vi "Process.vi"(8 "error in":errorcluster, 11 "Example Instrument UI":refnum<class "SR7220 UI.lvclass">) -> (0 "error out":errorcluster, 3 "Example Instrument UI out":refnum<class "SR7220 UI.lvclass">)   [LabVIEW 2016, in "SR7220 UI.lvclass"]
doc: "---------------------------------------------------------------\nJKI State Machine Objects™\nhttp://jki.net/state-machine-objects/\nCopyright (C) 2005-2015, JKI <info@jki.net>\nALL RIGHTS RESERVEDJKI State Machine Objects (SMO) 1.0.0.5\nJKI - JKI\nCopyright (c) 2016, JKI"
uses:
  SR7220 UI.lvclass
  C:/Program Files (x86)/National Instruments/LabVIEW 2016/vi.lib/JKI/JKI SMO/SMO/SMO.lvclass
  C:/Program Files (x86)/National Instruments/LabVIEW 2016/vi.lib/JKI/JKI SMO/SMO.UI/SMO.UI.lvclass
  Instrument.SR7270/Typedefs/SignalChannelConfig--Cluster.ctl
  Instrument.SR7270/Driver/Typedefs/VMODE--enum.ctl
  Instrument.SR7270/Driver/Typedefs/FLOAT--enum.ctl
  Instrument.SR7270/Driver/Typedefs/FET--enum.ctl
  Instrument.SR7270/Driver/Typedefs/LF--enum.ctl
  Instrument.SR7270/Driver/Typedefs/SEN-IMODE0--enum.ctl
  <vilib>/JKI/JKI SMO/SMO/Typedefs/Parent Call--Enum.ctl
  SR7220 UI.lvclass/SR7220 UI.ctl
  levylab_inst/lvsrc/SMOs/Instrument/Typedefs/PrivateEvents--Instrument.SendMessage.ctl
  <vilib>/JKI/JKI SMO/SMO.UI/SMO.UI.lvclass
  <vilib>/JKI/JKI SMO/SMO/SMO.lvclass
  levylab_inst/lvsrc/SMOs/Instrument/Instrument.lvclass
  Instrument.SR7270/Instrument.SR7270.lvclass
  Instrument.SR7270/Driver/SR7270 Drivers.lvclass
panel:
  out "Slide 4":dbl(slide) scale=0.0..10.0 scale format="%#_6p"
  out "Slide 3":dbl(slide) scale=0.0..10.0 scale format="%#_6p"
  out "Slide 2":dbl(slide) scale=0.0..10.0 scale format="%#_6p"
  out "Slide":dbl(slide) scale=0.0..10.0 scale format="%#_6p"
  in  "update time (ms)":u32=100
  out "Numeric 4":dbl
  out "Numeric 3":dbl
  out "Numeric 2":dbl
  out "Numeric":dbl
  in  "Display Type":enum16{"X", "Y", "MAG", "PHASE"}(ring)=enum."PHASE"
  in  "Display Type":enum16{"X", "Y", "MAG", "PHASE"}(ring)=enum."PHASE"
  in  "Display Type":enum16{"X", "Y", "MAG", "PHASE"}(ring)=enum."PHASE"
  in  "Display Type":enum16{"X", "Y", "MAG", "PHASE"}(ring)=enum."PHASE"
  in  "down":bool
  in  "up":bool
  in  "Sensitivity IMODE0":T1=enum."5 nV"
  in  "Signal Channel Config":T2={"Input Mode"=enum."Both Grounded", "Input Connector Shell"=enum."Float", "Input Device"=enum."FET", "Line Rejection Filter"=enum."Off"}
  in  "STOP":bool
  # "SMO UI Template"
  # "For instructions on how to use the JKI State Machine Objects, examples and video tutorials, visit:\nhttp://jki.net/state-machine-objects/\n\nJKI State Machine Objects™\nhttp://jki.net/state-machine-objects/\nCopyright (C) 2005-2015, JKI <info@jki.net>\nALL RIGHTS RESERVED"
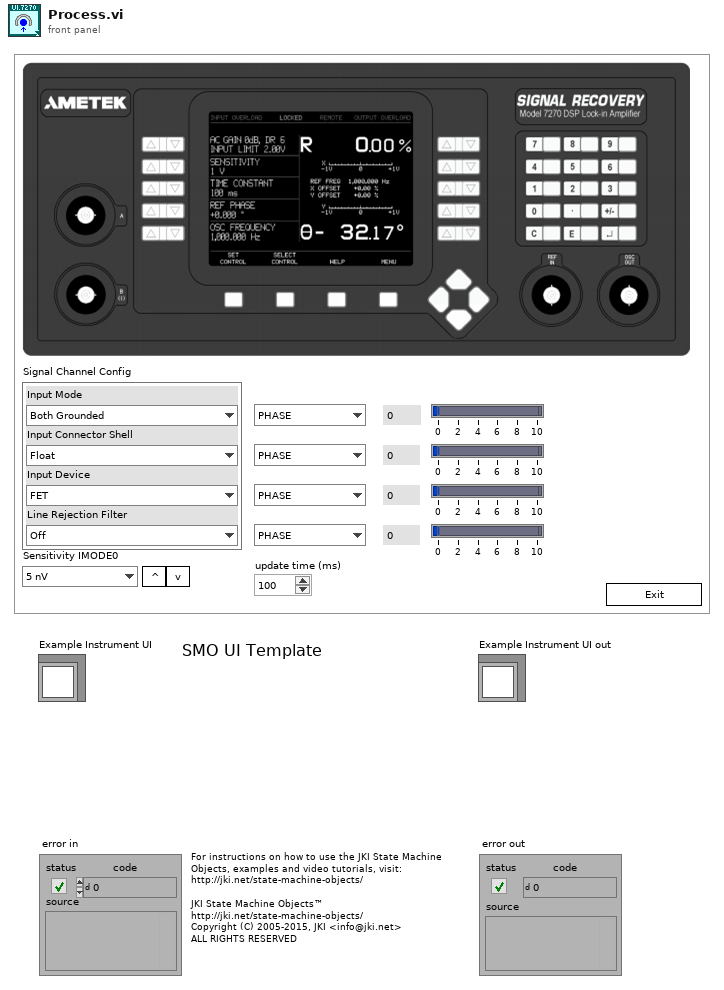
[diagram p1: front panel]
types:
  T1 = typedef "SR7270 Drivers.lvclass/SEN-IMODE0--enum.ctl" = enum16{"2 nV", "5 nV", "10 nV", "20 nV", "50 nV", "100 nV", "200 nV", "500 nV", "1 µV", "2 µV", "5 µV", "10 µV", "20 µV", "50 µV", "100 µV", "200 µV", "500 µV", "1 mV", "2 mV", "5 mV", "10 mV", "20 mV", "50 mV", "100 mV", "200 mV", "500 mV", "1 V"}
  T2 = typedef "Instrument.SR7270.lvclass/SignalChannelConfig--Cluster.ctl" = cluster{"Input Mode":T3, "Input Connector Shell":T4, "Input Device":T5, "Line Rejection Filter":T6}
  T3 = typedef "SR7270 Drivers.lvclass/VMODE--enum.ctl" = enum16{"Both Grounded", "A input only", "-B input only", "A-B differential"}
  T4 = typedef "SR7270 Drivers.lvclass/FLOAT--enum.ctl" = enum16{"Ground", "Float"}
  T5 = typedef "SR7270 Drivers.lvclass/FET--enum.ctl" = enum16{"Bipolar", "FET"}
  T6 = typedef "SR7270 Drivers.lvclass/LF--enum.ctl" = enum16{"Off", "60 Hz", "120 Hz", "60 & 120 Hz"}
  T7 = typedef "SMO.lvclass/Parent Call--Enum.ctl" = enum16{"Allows parent to run", "Does not request parent to run"}
  T8 = enum32{"invalid app kind", "Development System", "Run Time System", "Student Edition", "Embedded LabVIEW", "Evaluation", "Custom"}
  T9 = enum32{"Invalid", "Standard", "Closed", "Hidden", "Minimized", "Maximized"}
  T10 = typedef "Instrument.lvclass/PrivateEvents--Instrument.SendMessage.ctl" = cluster{"Message":cluster{"Command":string, "Data":variant}, "Message ID":u32}
  T11 = typedef "Instrument.lvclass/PublicEvents--Instrument.get all.ctl" = variant
  T12 = cluster{"Core":cluster{"Current VI Reference":refnum<vi>, "Close Panel on Exit?":bool, "error":errorcluster}, "Self Reference":refnum<class "SR7220 UI.lvclass">, "Instrument":refnum<class "Instrument.lvclass">, "getAll":variant, "Data":variant}
  T13 = cluster{"Current VI Reference":refnum<vi>, "Close Panel on Exit?":bool, "error":errorcluster}
  T14 = typedef "SMO.lvclass/Protected Events.ctl" = cluster{"StopProcesses":refnum<user-event>, "AbortProcesses":refnum<user-event>, "Config Changed":refnum<user-event>, "Dependency":refnum<user-event>}
  T15 = typedef "Instrument.lvclass/PublicEvents--Cluster.ctl" = cluster{"get all":refnum<user-event>}
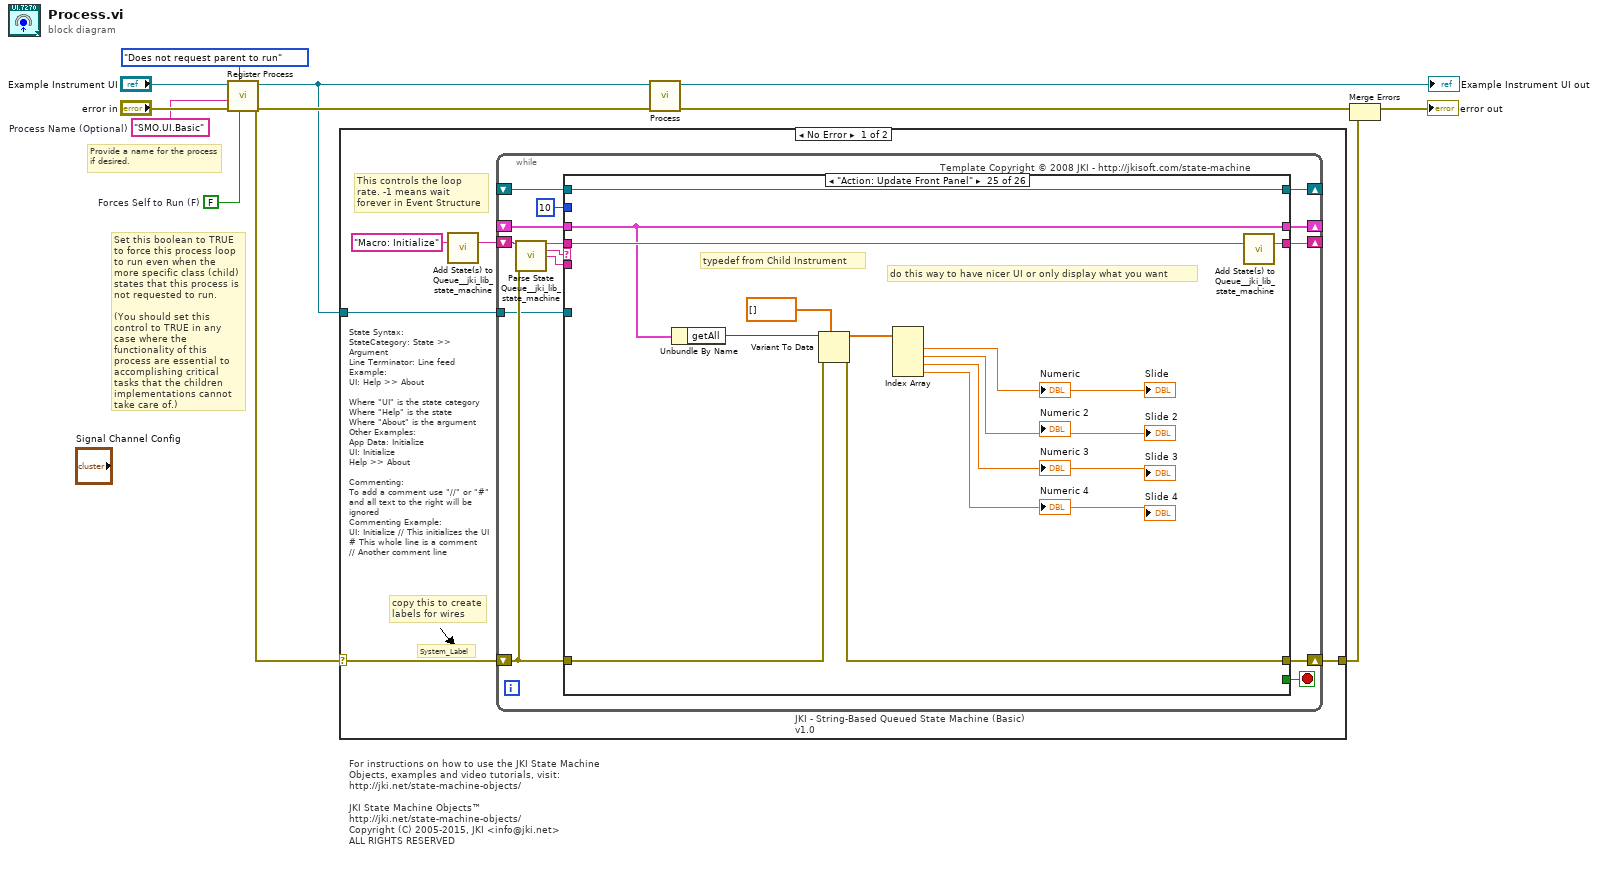
[diagram p0: block diagram]
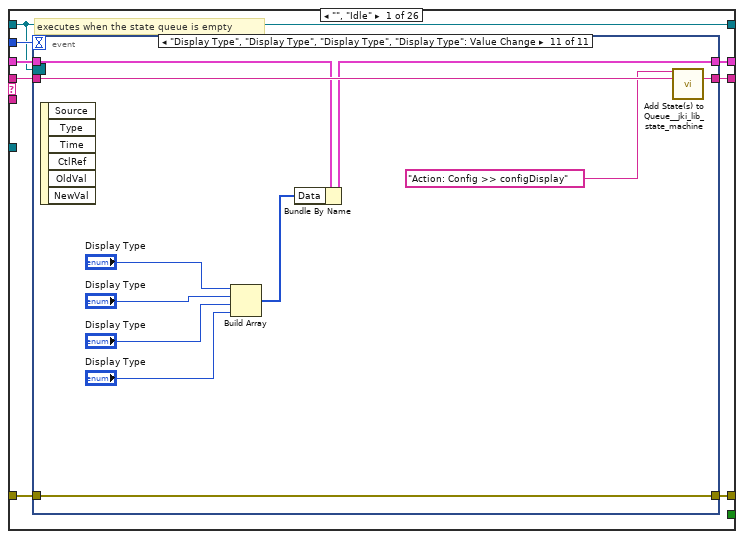
[diagram p2: hidden frame]
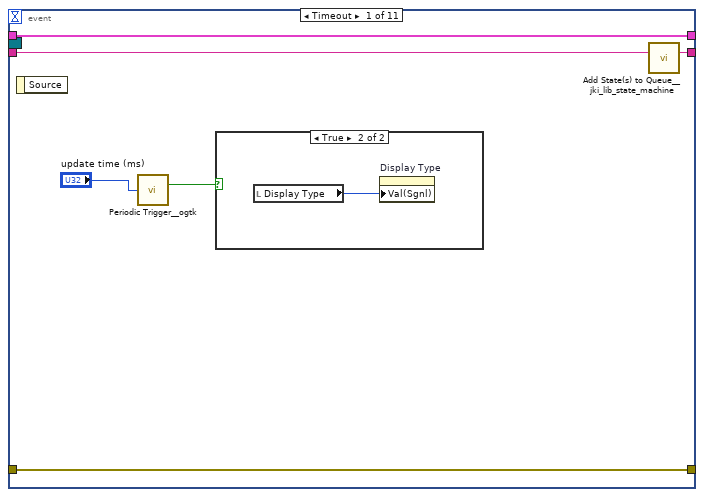
[diagram p3: hidden frame]
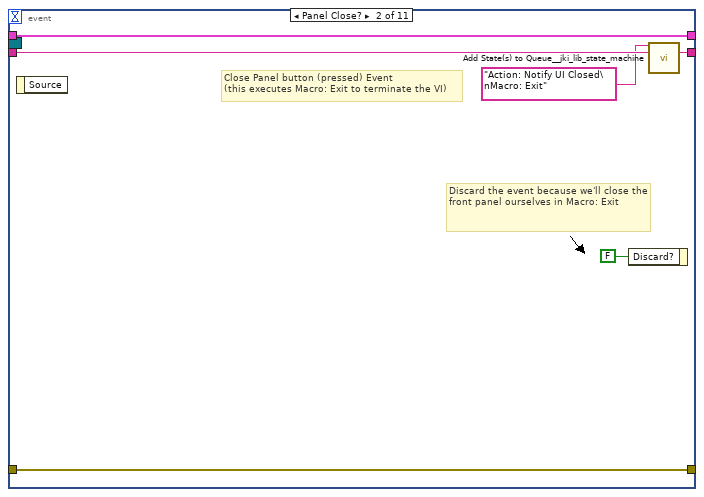
[diagram p5: hidden frame]
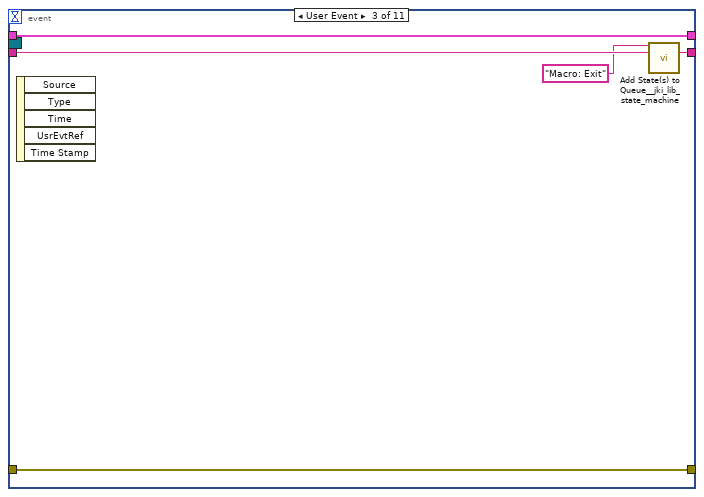
[diagram p6: hidden frame]
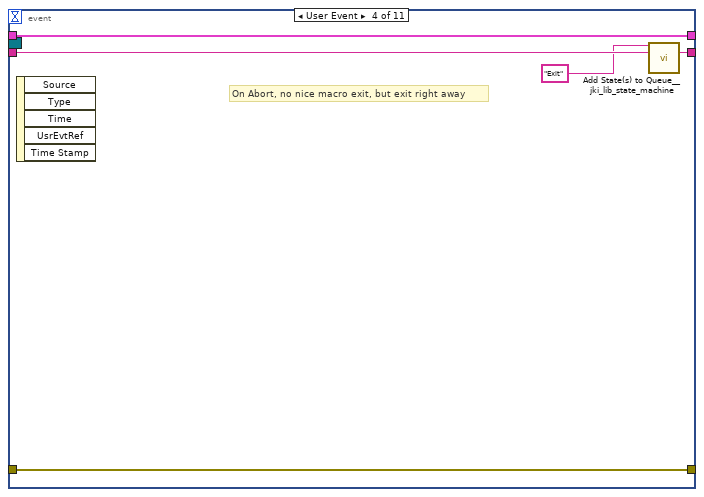
[diagram p7: hidden frame]
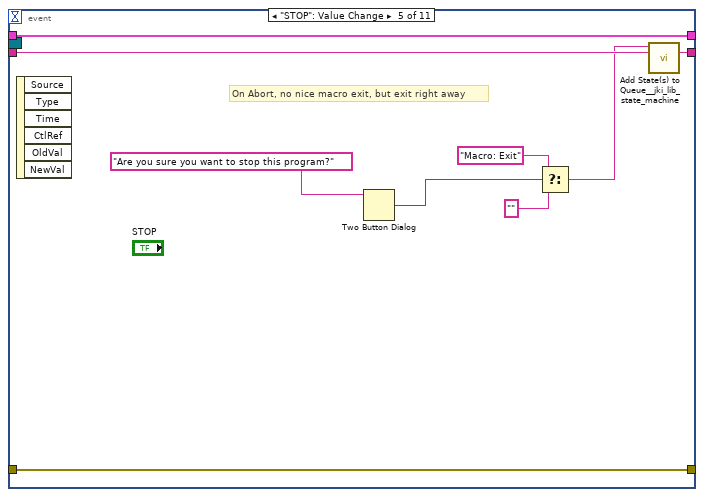
[diagram p8: hidden frame]
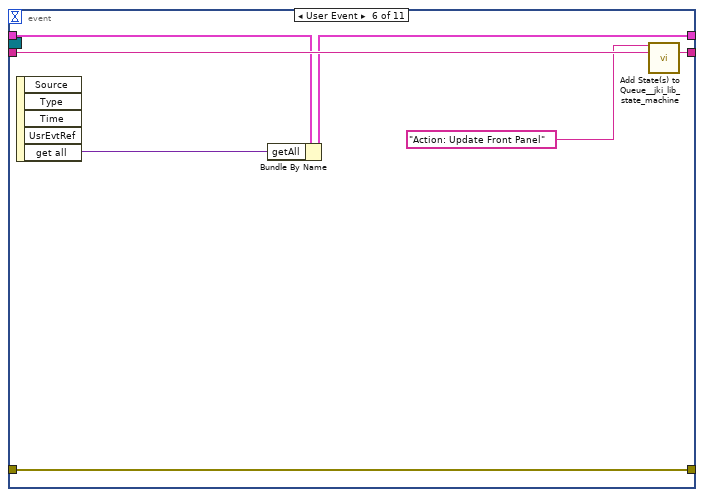
[diagram p9: hidden frame]
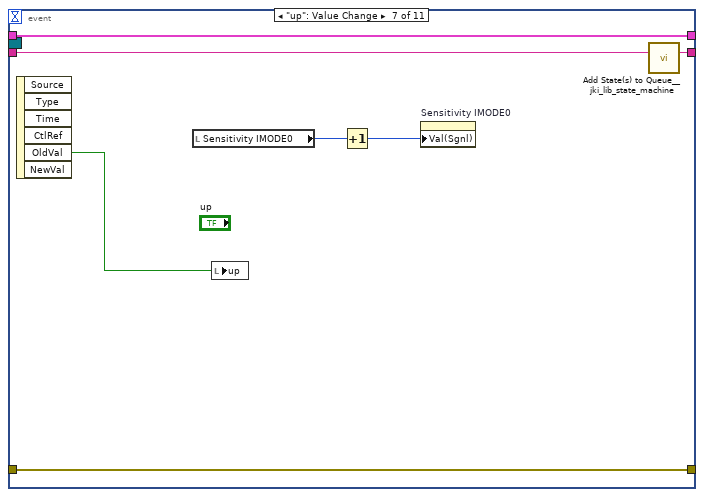
[diagram p10: hidden frame]
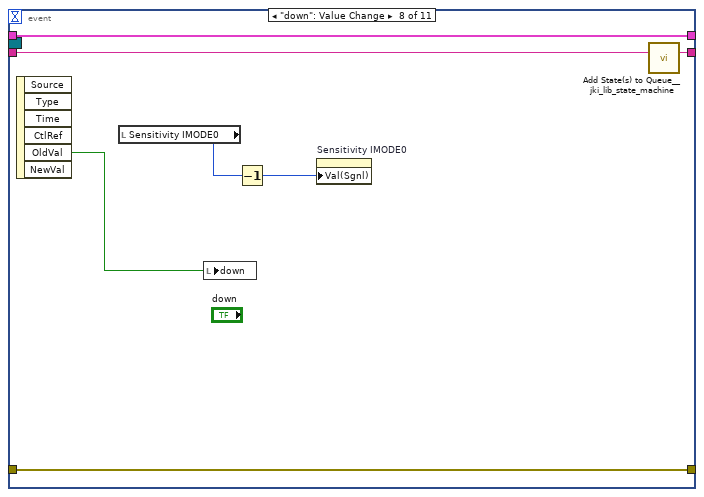
[diagram p11: hidden frame]
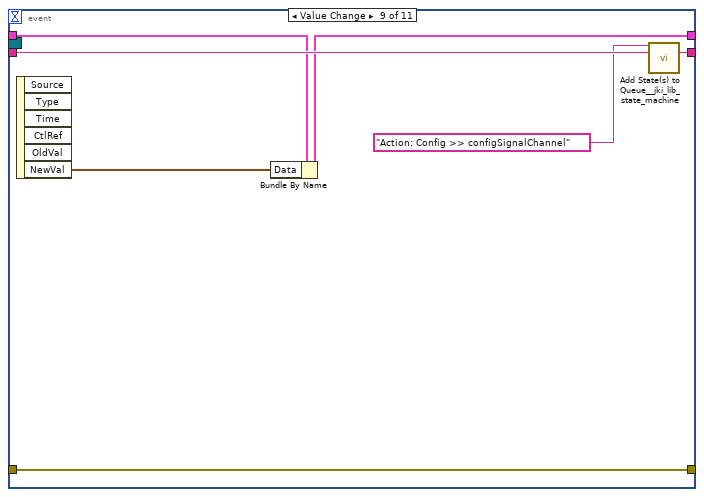
[diagram p12: hidden frame]
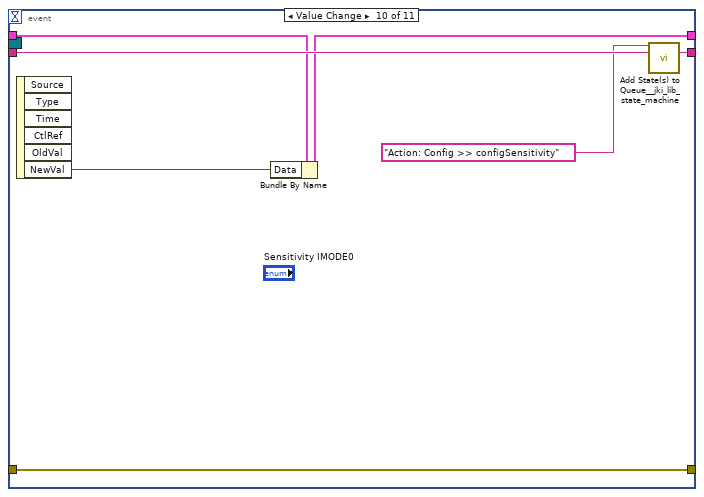
[diagram p13: hidden frame]
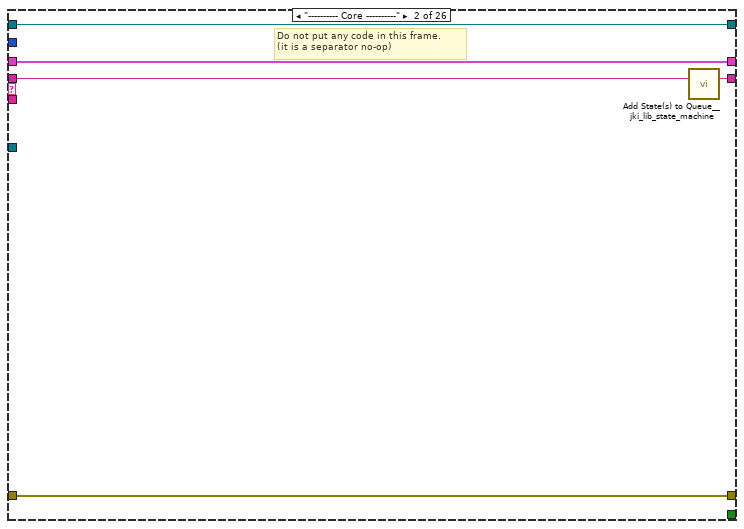
[diagram p14: hidden frame]
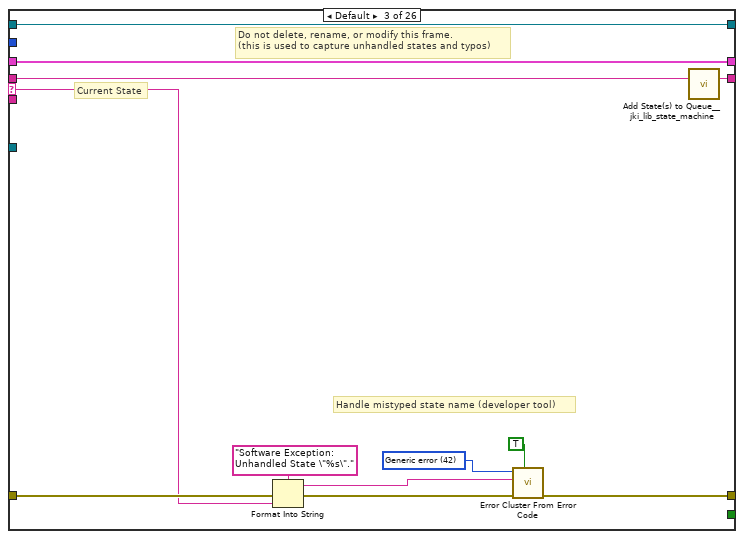
[diagram p15: hidden frame]
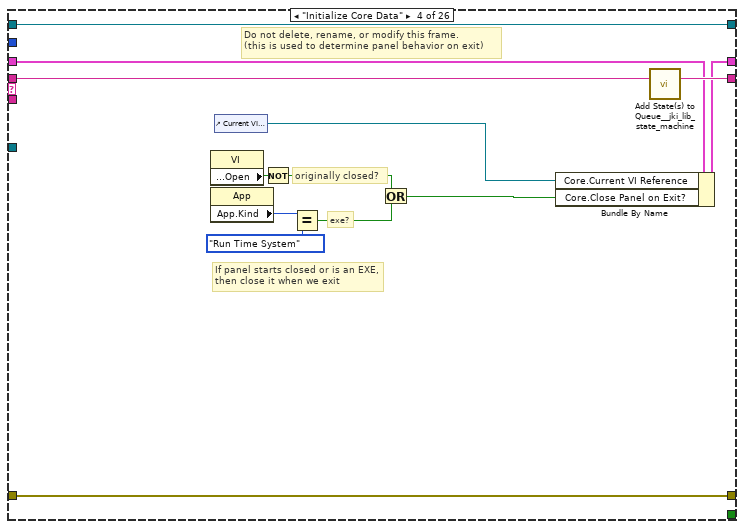
[diagram p16: hidden frame]
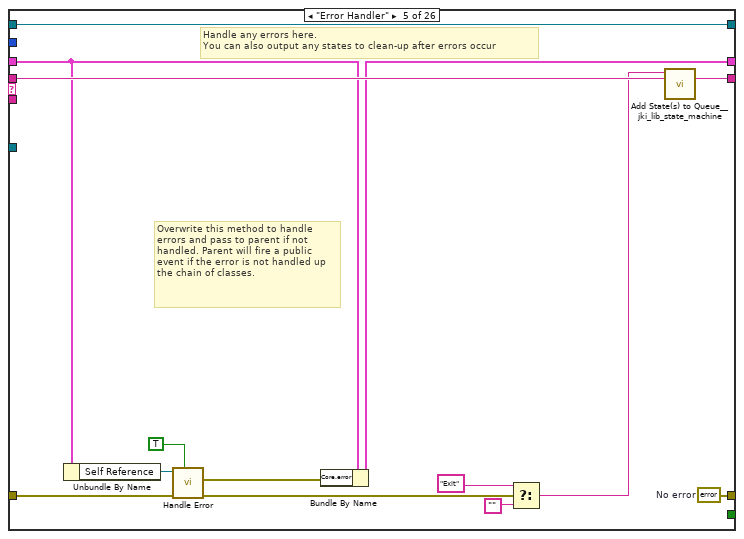
[diagram p17: hidden frame]
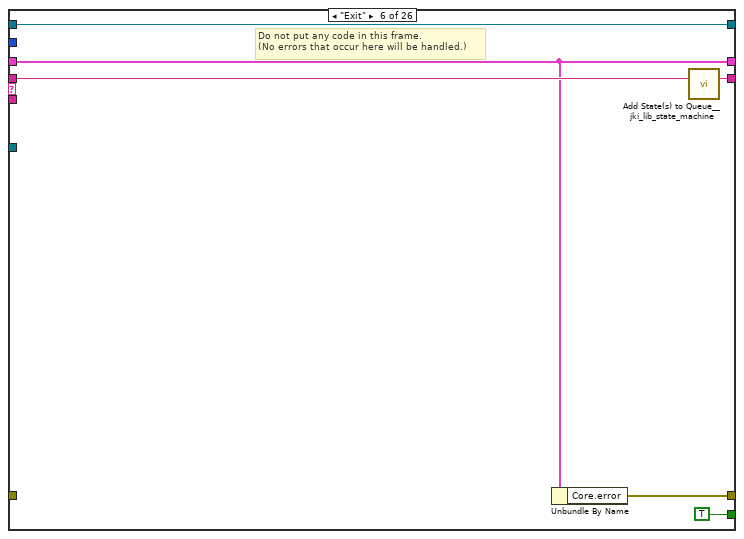
[diagram p18: hidden frame]
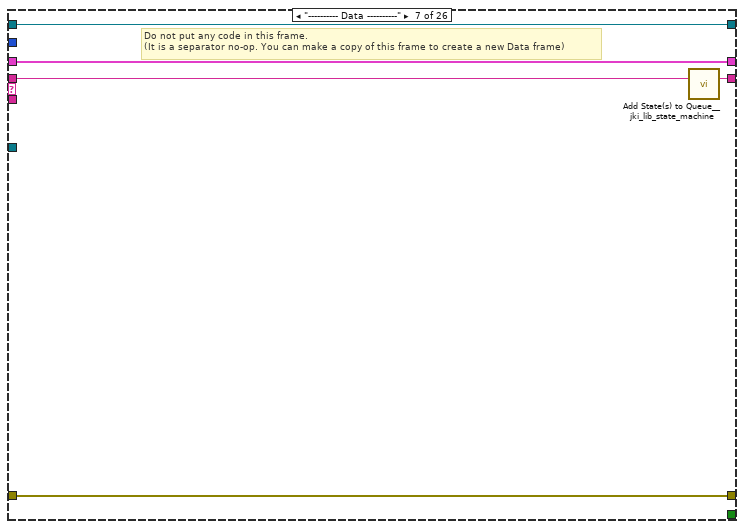
[diagram p19: hidden frame]
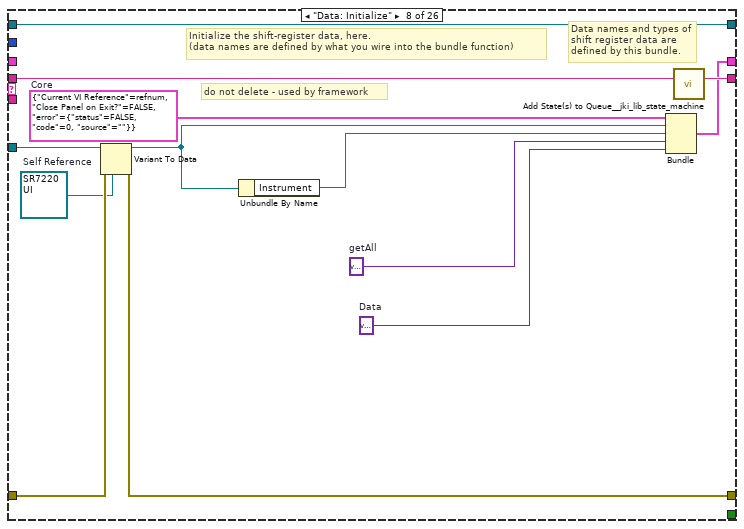
[diagram p20: hidden frame]
diagram:
  w2 = FALSE  # Forces Self to Run (F)
  w1 = "SMO.UI.Basic"  # Process Name (Optional)
  # "Provide a name for the process\nif desired."
  # "Set this boolean to TRUE to force this process loop to run even when the more specific class (child) states that this process is not requested to run.\n\n(You should set this control to TRUE in any case where the functionality of this process are essential to accomplishing critical tasks that the children implementations cannot take care of.)"
  # "For instructions on how to use the JKI State Machine Objects, examples and video tutorials, visit:\nhttp://jki.net/state-machine-objects/\n\nJKI State Machine Objects™\nhttp://jki.net/state-machine-objects/\nCopyright (C) 2005-2015, JKI <info@jki.net>\nALL RIGHTS RESERVED"
  n1 = call <vilib>:"Register Process.vi"("Forces Self to Run (F)"=w2, "Parent Call"=Parent_Call--Enum."Does not request parent to run", "error in (no error)"="error in", "Process Name (optional)"=w1, "SMO"="Example Instrument UI") -> ("error out"=w8:errorcluster, "SMO out"=w7:refnum<class "SR7220 UI.lvclass">)  [unwired: 5 in]
  n2 = case shown="No Error" w8 {
    selector: w8 -> [w13 w367]
    tunnel: w7 -> [w14 _]
    tunnel: [w12 w367] -> w4
    frame No Error {
      # "State Syntax:\nStateCategory: State >> Argument\nLine Terminator: Line feed\nExample:\nUI: Help >> About\n\nWhere \"UI\" is the state category\nWhere \"Help\" is the state\nWhere \"About\" is the argument\nOther Examples:\nApp Data: Initialize\nUI: Initialize\nHelp >> About\n\nCommenting:\nTo add a comment use \"//\" or \"#\" and all text to the right will be ignored\nCommenting Example:\nUI: Initialize // This initializes the UI\n# This whole line is a comment\n// Another comment line"
      # "copy this to create labels for wires"
      # "This controls the loop rate. -1 means wait forever in Event Structure"
      # "System_Label"
      n3 = call <vilib>:"Add State(s) to Queue__jki_lib_state_machine.vi"("State(s) in (\"\")"="Macro: Initialize") -> ("States Out"=w16:string)  [unwired: 14 in]
      n4 = while "JKI - String-Based Queued State Machine (Basic) v1.0" {
        shift-right: [w23] -> _
        shift-left: _ -> [w22]
        shift-right: [w26] -> w12
        shift-left: w13 -> [w20]
        shift-right: [w25] -> _
        shift-left: w16 -> [w27]
        tunnel: w14 -> [w19]
        shift-right: [w18] -> _
        shift-left: _ -> [w17]
        stop <- w24 stop-if-true
        # "Template Copyright © 2008 JKI - http://jkisoft.com/state-machine"
        n5 = call <vilib>:"Parse State Queue__jki_lib_state_machine.vi"("State Queue"=w27, "Error In (no error)"=w20) -> ("Remaining States"=w29:string, "Current State"=w30:string, "Arguments"=w28:string)  [unwired: 11 in]
        n6 = case shown="\"Action: Update Front Panel\"" w30 {
          selector: w30 -> [_ _ w123 _ _ _ _ _ _ _ _ _ _ _ _ _ _ _ _ _ _ _ _ _ _ _]
          tunnel: w29 -> [w38 w121 w127 w146 w160 w166 w171 w184 w191 w196 w203 w210 w226 w258 w267 w281 w286 w297 w304 w309 w322 w328 w335 w342 w355 w366]
          tunnel: w28 -> [_ _ _ _ _ _ _ _ _ _ _ w204 w220 _ _ _ _ _ _ _ _ _ _ _ _ w357]
          tunnel: w22 -> [w36 w118 w125 w137 w149 w162 w168 _ w186 w193 w201 w208 w222 w255 w263 w272 w283 w294 w299 w306 w320 w326 w331 w338 w352 w363]
          tunnel: [w35 w119 w129 w143 w151 w161 w169 w180 w187 w194 w198 w205 w223 w256 w265 w279 w284 w288 w300 w307 w315 w323 w332 w336 w349 w361] -> w26
          tunnel: w20 -> [w34 w119 w128 w143 w156 _ w169 w181 w188 w194 w199 w206 w224 w256 w265 w279 w284 w289 w301 w307 w317 w324 w332 w337 w350 w362]
          tunnel: [w37 w120 w126 w145 w159 w165 w170 w183 w190 w195 w202 w209 w225 w257 w266 w280 w285 w296 w303 w308 w321 w327 w334 w341 w354 w365] -> w25
          tunnel: [_ _ _ _ _ TRUE _ _ _ _ _ _ _ _ _ _ _ _ _ _ _ _ _ _ _ _] -> w24
          tunnel: [w33 w118 w125 w144 w148 w162 w168 w182 w186 w193 w201 w208 w222 w255 w263 w272 w283 w294 w299 w306 w320 w326 w330 w338 w352 w363] -> w23
          tunnel: 10 ("Timeout") -> [w32 _ _ _ _ _ _ _ _ _ _ _ _ _ _ _ _ _ _ _ _ _ _ _ _ _]
          tunnel: w19 -> [_ _ _ _ _ _ _ w178 _ _ _ _ _ _ _ _ _ _ _ _ _ _ _ _ _ _]
          tunnel: [w31 w117 w122 w134 w158 w163 w167 w177 w185 w192 w200 w207 w219 w254 w264 w273 w282 w295 w302 w305 w319 w325 w333 w340 w353 w364] -> w18
          tunnel: w17 -> [w31 w117 w122 w134 w158 w163 w167 w177 w185 w192 w200 w207 w219 w254 w264 w273 w282 w295 w302 w305 _ w325 w333 w340 w353 w364]
          frame "", "Idle" {
            # "executes when the state queue is empty"
            n7 = event shown="[10] \"Display Type\", \"Display Type\", \"Display Type\", \"Display Type\": Value Change" {
              selector: w31 -> [_ _ _ _ _ _ _ _ _ _ _]
              dyn-events: _ -> [_ _ _ _ _ _ _ _ _ _ _]
              timeout: w32 -> [_ _ _ _ _ _ _ _ _ _ _]
              tunnel: w38 -> [w44 w51 w56 w61 w70 w77 w84 w91 w98 w105 w116]
              tunnel: [w43 w50 w55 w60 w69 w76 w83 w90 w97 w104 w115] -> w37
              tunnel: w36 -> [w41 w47 w53 w58 w67 w72 w81 w88 w94 w101 w112]
              tunnel: [w42 w46 w54 w59 w68 w74 w82 w89 w95 w102 w113] -> w35
              tunnel: w34 -> [w42 w46 w54 w59 w68 w74 w82 w89 w95 w102 w113]
              tunnel: [w41 w47 w53 w58 w67 w71 w81 w88 w93 w100 w111] -> w33
              event Timeout {
                n8 = event-data() -> ()  [unwired: 1 in, 1 out]
                n9 = call <userlib>:"Periodic Trigger__ogtk.vi"("time (ms)"="update time (ms)") -> ("Triggered"=w40:bool)  [unwired: 12 in, 2 out]
                n10 = case shown="True" w40 {
                  frame False {
                  }
                  frame True {
                    n11 = local read "Display Type"() -> (w45:enum16{"X", "Y", "MAG", "PHASE"})
                    n12 = property on="Display Type" class="Enum (strict)"("Val(Sgnl)"=w45) -> ()  [unwired: 2 in, 2 out]
                  }
                }
                n13 = call <vilib>:"Add State(s) to Queue__jki_lib_state_machine.vi"("State(s) in (\"\")"=w44) -> ("States Out"=w43:string)  [unwired: 14 in]
              }
              event Panel Close? {
                # "Discard the event because we'll close the front panel ourselves in Macro: Exit"
                # "Close Panel button (pressed) Event\n(this executes Macro: Exit to terminate the VI)"
                n14 = event-data() -> ()  [unwired: 1 in, 1 out]
                n15 = event-data("Discard?"=FALSE) -> ()  [unwired: 1 in, 1 out]
                n16 = call <vilib>:"Add State(s) to Queue__jki_lib_state_machine.vi"("State(s) in Front (\"\")"="Action: Notify UI Closed\nMacro: Exit", "State(s) in (\"\")"=w51) -> ("States Out"=w50:string)  [unwired: 13 in]
              }
              event User Event {
                n17 = event-data() -> ()  [unwired: 1 in, 5 out]
                n18 = call <vilib>:"Add State(s) to Queue__jki_lib_state_machine.vi"("State(s) in Front (\"\")"="Macro: Exit", "State(s) in (\"\")"=w56) -> ("States Out"=w55:string)  [unwired: 13 in]
              }
              event User Event {
                # "On Abort, no nice macro exit, but exit right away"
                n19 = event-data() -> ()  [unwired: 1 in, 5 out]
                n20 = call <vilib>:"Add State(s) to Queue__jki_lib_state_machine.vi"("State(s) in Front (\"\")"="Exit", "State(s) in (\"\")"=w61) -> ("States Out"=w60:string)  [unwired: 13 in]
              }
              event "STOP": Value Change {
                # "On Abort, no nice macro exit, but exit right away"
                n21 = event-data() -> ()  [unwired: 1 in, 6 out]
                n22 = Two Button Dialog(message="Are you sure you want to stop this program?") -> (T button?=w66:bool)  [unwired: 2 in]
                n23 = Select(t="Macro: Exit", s=w66, f="") -> (s? t:f=w62:string)
                n24 = call <vilib>:"Add State(s) to Queue__jki_lib_state_machine.vi"("State(s) in Front (\"\")"=w62, "State(s) in (\"\")"=w70) -> ("States Out"=w69:string)  [unwired: 13 in]
              }
              event User Event {
                n25 = event-data() -> ("get all"=w73:T11)  [unwired: 1 in, 4 out]
                n26 = Bundle By Name(cluster=w72, "getAll"=w73) -> (w71:T12)
                n27 = call <vilib>:"Add State(s) to Queue__jki_lib_state_machine.vi"("State(s) in Front (\"\")"="Action: Update Front Panel", "State(s) in (\"\")"=w77) -> ("States Out"=w76:string)  [unwired: 13 in]
              }
              event "up": Value Change {
                n28 = event-data() -> ("OldVal"=w78:bool)  [unwired: 1 in, 5 out]
                n29 = local read "Sensitivity IMODE0"() -> (w80:T1)
                n30 = local write "up"(w78) -> ()
                n31 = Increment(x=w80) -> (x+1=w79:T1)
                n32 = property on="Sensitivity IMODE0" class="Enum (strict)"("Val(Sgnl)"=w79) -> ()  [unwired: 2 in, 2 out]
                n33 = call <vilib>:"Add State(s) to Queue__jki_lib_state_machine.vi"("State(s) in (\"\")"=w84) -> ("States Out"=w83:string)  [unwired: 14 in]
              }
              event "down": Value Change {
                n34 = event-data() -> ("OldVal"=w85:bool)  [unwired: 1 in, 5 out]
                n35 = local read "Sensitivity IMODE0"() -> (w87:T1)
                n36 = local write "down"(w85) -> ()
                n37 = Decrement(x=w87) -> (x-1=w86:T1)
                n38 = property on="Sensitivity IMODE0" class="Enum (strict)"("Val(Sgnl)"=w86) -> ()  [unwired: 2 in, 2 out]
                n39 = call <vilib>:"Add State(s) to Queue__jki_lib_state_machine.vi"("State(s) in (\"\")"=w91) -> ("States Out"=w90:string)  [unwired: 14 in]
              }
              event Value Change {
                n40 = event-data() -> ("NewVal"=w92:T2)  [unwired: 1 in, 5 out]
                n41 = Bundle By Name(cluster=w94, "Data"=w92) -> (w93:T12)
                n42 = call <vilib>:"Add State(s) to Queue__jki_lib_state_machine.vi"("State(s) in Front (\"\")"="Action: Config >> configSignalChannel", "State(s) in (\"\")"=w98) -> ("States Out"=w97:string)  [unwired: 13 in]
              }
              event Value Change {
                n43 = event-data() -> ("NewVal"=w99:T1)  [unwired: 1 in, 5 out]
                n44 = Bundle By Name(cluster=w101, "Data"=w99) -> (w100:T12)
                n45 = call <vilib>:"Add State(s) to Queue__jki_lib_state_machine.vi"("State(s) in Front (\"\")"="Action: Config >> configSensitivity", "State(s) in (\"\")"=w105) -> ("States Out"=w104:string)  [unwired: 13 in]
              }
              event "Display Type", "Display Type", "Display Type", "Display Type": Value Change {
                n46 = event-data() -> ()  [unwired: 1 in, 6 out]
                n47 = Build Array("Display Type", "Display Type", "Display Type", "Display Type") -> (w106:enum16{"X", "Y", "MAG", "PHASE"}[])
                n48 = Bundle By Name(cluster=w112, "Data"=w106) -> (w111:T12)
                n49 = call <vilib>:"Add State(s) to Queue__jki_lib_state_machine.vi"("State(s) in Front (\"\")"="Action: Config >> configDisplay", "State(s) in (\"\")"=w116) -> ("States Out"=w115:string)  [unwired: 13 in]
              }
            }
          }
          frame "---------- Core ----------" {
            # "Do not put any code in this frame.\n(it is a separator no-op)"
            n50 = call <vilib>:"Add State(s) to Queue__jki_lib_state_machine.vi"("State(s) in (\"\")"=w121) -> ("States Out"=w120:string)  [unwired: 14 in]
          }
          frame Default {
            w132 = 42 items=["No error", "Argument error", "Memory is full", "Out of zone", "End of file", "File already open", "Generic file I/O error", "File not found", "File permission error", "Disk is full", "Duplicate path", "Too many files open", "System feature not enabled", "Resource file not found", "Cannot add resource", "Resource not found", "Image not found", "Image memory error", "Pen does not exist", "Config type invalid", "Config token not found", "Config parse error", "Config memory error", "Bad external code format", "Bad external code offset", "External code not present", "Null window", "Destroy window error", "Null menu", "Print aborted", "Bad print record", "Print driver error", "Windows error during printing", "Memory error during printing", "Print dialog error", "Generic print error", "Invalid device refnum", "Device not found", "Device parameter error", "Device unit error", "Cannot open device", "Device call aborted", "Generic error", "Cancelled by user", "Object ID too low", "Object ID too high", "Object not in heap", "Unknown heap", "Unknown object (invalid DefProc)", "Unknown object (DefProc not in table)", "Message out of range", "Invalid (null) method", "Unknown message", "Manager call not supported", "Bad address", "Network operation in progress", "Network operation timed out", "Connection is busy", "Network attribute not supported", "Network error", "Address in use", "System out of memory", "Connection aborted", "Connection refused", "Not connected", "Already connected", "Connection closed", "Initialization error (interapplication manager)", "Bad occurrence", "Wait on unbound occurrence handler", "Occurrence queue overflow", "Datalog type conflict", "Unused", "Unrecognized type (interapplication manager)", "Memory corrupt", "Failed to make temporary DLL", "Old CIN version", "Drag socket not found", "Failed to load drop-object", "Failed to register OLE object", "Failed to release OLE object", "Format specifier type mismatch", "Unknown format specifier", "Too few format specifiers", "Too many format specifiers", "Scan failed", "Newer CIN version", "Error converting to variant", "Runtime menu error", "Password tampered", "Variant attribute not found", "Incompatible variant data type", "Event data is not available", "Event Store is not present", "Occurrence is not found", "Event Queue is not created", "Event info is not available", "Refnum passed is NULL", "Error retrieving Class GUID", "Error retrieving CoClass GUID", "Error retrieving TypeLib GUID.", "Bad built application magic bytes.", "Specific driver is different from the specific driver associated with the Logical Name.", "There is no session opened to the class driver.", "Max Error", "MAX - Error with config objects", "MAX - Error loading configuration", "MAX - Group not supported"]
            # "Current State"
            # "Do not delete, rename, or modify this frame.\n(this is used to capture unhandled states and typos)"
            # "Handle mistyped state name (developer tool)"
            n51 = Format Into String(format string="Software Exception: Unhandled State \"%s\"." ("message"), error in=w128, w123) -> (resulting string=w131:string, error out=w130:errorcluster)  [unwired: 1 in]
            n52 = call <vilib>:"Error Cluster From Error Code.vi"("show call chain? (False)"=TRUE, "error in (no error)"=w130, "error message (\"\")"=w131, "error code (0)"=w132) -> ("error out"=w129:errorcluster)  [unwired: 5 in]
            n53 = call <vilib>:"Add State(s) to Queue__jki_lib_state_machine.vi"("State(s) in (\"\")"=w127) -> ("States Out"=w126:string)  [unwired: 14 in]
          }
          frame "Initialize Core Data" {
            # "Do not delete, rename, or modify this frame.\n(this is used to determine panel behavior on exit)"
            # "originally closed?"
            # "exe?"
            # "If panel starts closed or is an EXE, then close it when we exit"
            n54 = property class="VI"() -> ("Front Panel.Open"=w142:bool)  [unwired: 2 in, 2 out]
            n55 = property class="App"() -> ("App.Kind"=w141:T8)  [unwired: 2 in, 2 out]
            n56 = control-ref of="Current VI Reference"() -> (w135:refnum<vi>)
            n57 = Not(x=w142) -> (.not. x?=w139:bool)
            n58 = Equal?(x=w141, y=T8."Run Time System" ("Application:Kind")) -> (x = y?=w138:bool)
            n59 = Or(x=w139, y=w138) -> (x .or. y?=w136:bool)
            n60 = Bundle By Name(cluster=w137, "Core.Current VI Reference"=w135, "Core.Close Panel on Exit?"=w136) -> (w144:T12)
            n61 = call <vilib>:"Add State(s) to Queue__jki_lib_state_machine.vi"("State(s) in (\"\")"=w146) -> ("States Out"=w145:string)  [unwired: 14 in]
          }
          frame "Error Handler" {
            w151 = errorcluster {"status"=FALSE, "code"=0, "source"=""}  # No error
            # "Overwrite this method to handle errors and pass to parent if not handled. Parent will fire a public event if the error is not handled up the chain of classes."
            # "Handle any errors here.\nYou can also output any states to clean-up after errors occur"
            n62 = Unbundle By Name(w149) -> ("Self Reference"=w157:refnum<class "SR7220 UI.lvclass">)
            n63 = call-dynamic "Handle Error.vi"("Stop on Unhandled Error (T)"=TRUE, "error in"=w156, "SMO"=w157) -> ("handling error"=w152:errorcluster, "Unhandled error"=w150:errorcluster)  [unwired: 6 in, 1 out]
            n64 = Bundle By Name(cluster=w149, "Core.error"=w150) -> (w148:T12)
            n65 = Select(t="Exit", s=w152, f="") -> (s? t:f=w153:string)
            n66 = call <vilib>:"Add State(s) to Queue__jki_lib_state_machine.vi"("State(s) in Front (\"\")"=w153, "State(s) in (\"\")"=w160) -> ("States Out"=w159:string)  [unwired: 13 in]
          }
          frame "Exit" {
            # "Do not put any code in this frame.\n(No errors that occur here will be handled.)"
            n67 = Unbundle By Name(w162) -> ("Core.error"=w161:errorcluster)
            n68 = call <vilib>:"Add State(s) to Queue__jki_lib_state_machine.vi"("State(s) in (\"\")"=w166) -> ("States Out"=w165:string)  [unwired: 14 in]
          }
          frame "---------- Data ----------" {
            # "Do not put any code in this frame.\n(It is a separator no-op. You can make a copy of this frame to create a new Data frame)"
            n69 = call <vilib>:"Add State(s) to Queue__jki_lib_state_machine.vi"("State(s) in (\"\")"=w171) -> ("States Out"=w170:string)  [unwired: 14 in]
          }
          frame "Data: Initialize" {
            w172 = variant  # Data
            w173 = variant  # getAll
            w176 = T13 {"Current VI Reference"=refnum, "Close Panel on Exit?"=FALSE, "error"={"status"=FALSE, "code"=0, "source"=""}}  # Core
            w179 = refnum<class "SR7220 UI.lvclass"> refnum  # Self Reference
            # "do not delete - used by framework"
            # "Data names and types of shift register data are defined by this bundle."
            # "Initialize the shift-register data, here.\n(data names are defined by what you wire into the bundle function)"
            n70 = Variant To Data(error in=w181, type=w179, Variant=w178) -> (data=w175:refnum<class "SR7220 UI.lvclass">, error out=w180:errorcluster)
            n71 = Unbundle By Name(w175) -> ("Instrument"=w174:refnum<class "Instrument.lvclass">)
            n72 = Bundle("Core"=w176, "Self Reference"=w175, "Instrument"=w174, "getAll"=w173, "Data"=w172) -> (w182:T12)  [unwired: 1 in]
            n73 = call <vilib>:"Add State(s) to Queue__jki_lib_state_machine.vi"("State(s) in (\"\")"=w184) -> ("States Out"=w183:string)  [unwired: 14 in]
          }
          frame "Data: Cleanup" {
            # "Cleanup any data and references, here.\n(this is called automatically, by the Macro: Exit)"
            n74 = Unbundle By Name(w186) -> ("Core.Current VI Reference"=w189:refnum<vi>)
            n75 = Close Reference(reference=w189, error in (no error)=w188) -> (error out=w187:errorcluster)
            n76 = call <vilib>:"Add State(s) to Queue__jki_lib_state_machine.vi"("State(s) in (\"\")"=w191) -> ("States Out"=w190:string)  [unwired: 14 in]
          }
          frame "---------- UI ----------" {
            # "Do not put any code in this frame.\n(It is a separator no-op. You can make a copy of this frame to create a new UI frame)"
            n77 = call <vilib>:"Add State(s) to Queue__jki_lib_state_machine.vi"("State(s) in (\"\")"=w196) -> ("States Out"=w195:string)  [unwired: 14 in]
          }
          frame "UI: Initialize" {
            # "size window to decoration box on front panel"
            # "Initialize the User Interface, here.\n(this is called automatically, by the Macro: Init)"
            n78 = invoke on="STOP" class="Bool (strict)" method="Reinit To Default"() -> ()  [unwired: 3 in, 3 out]
            n79 = invoke on="down" class="Bool (strict)" method="Reinit To Default"() -> ()  [unwired: 3 in, 3 out]
            n80 = call <userlib>:"Fit VI window to Largest Dec__ogtk.vi"("error in (no error)"=w199, "border spacing (2 px)"=0) -> ("error out"=w198:errorcluster)  [unwired: 4 in, 1 out]
            n81 = invoke on="up" class="Bool (strict)" method="Reinit To Default"() -> ()  [unwired: 3 in, 3 out]
            n82 = call <vilib>:"Add State(s) to Queue__jki_lib_state_machine.vi"("State(s) in (\"\")"=w203) -> ("States Out"=w202:string)  [unwired: 14 in]
          }
          frame "UI: Cursor Set" {
            # "Argument"
            # "Initialize the User Interface, here.\n(this is called automatically, by the Macro: Init)"
            n83 = disable-structure shown="Default" {
              disable-tunnel: w206 -> [w211 w214]
              disable-tunnel: [w211 w213] -> w205
              disable-tunnel: w204 -> [_ w212]
              frame condition #0 {
              }
              frame condition #1 (active) {
                n84 = case shown="\"Busy\"" w212 {
                  tunnel: w214 -> [w216 w218]
                  tunnel: [w215 w217] -> w213
                  frame "Idle", Default {
                    n85 = call <vilib>:"Unset Busy.vi"("error in (no error)"=w216) -> ("error out"=w215:errorcluster)  [unwired: 10 in]
                  }
                  frame "Busy" {
                    n86 = call <vilib>:"Set Busy.vi"("error in (no error)"=w218) -> ("error out"=w217:errorcluster)  [unwired: 9 in, 1 out]
                  }
                }
              }
            }
            n87 = call <vilib>:"Add State(s) to Queue__jki_lib_state_machine.vi"("State(s) in (\"\")"=w210) -> ("States Out"=w209:string)  [unwired: 14 in]
          }
          frame "UI: Front Panel State" {
            # "Argument"
            # "Set Front Panel Open or Closed\n(Usage: \"UI: Front Panel State >> Open|Close\")"
            n88 = Unbundle By Name(w222) -> ("Core.Current VI Reference"=w221:refnum<vi>)
            n89 = disable-structure shown="Default" {
              disable-tunnel: w224 -> [w230 w253]
              disable-tunnel: [w229 w253] -> w223
              disable-tunnel: w221 -> [w228 _]
              disable-tunnel: w220 -> [w227 _]
              frame condition #0 (active) {
                n90 = case shown="\"Close\"" w227 {
                  tunnel: w230 -> [w234 w247]
                  tunnel: [w236 w248] -> w229
                  tunnel: w228 -> [w235 w245]
                  frame "Open", Default {
                    n91 = property class="VI"(reference=w235, error in=w234) -> (reference out=w232:refnum<vi>, error out=w233:errorcluster, "FP.State"=w231:T9)
                    n92 = case shown="\"Closed\"" w231 {
                      tunnel: [w239 w242] -> w236
                      tunnel: w233 -> [w238 w242]
                      tunnel: w232 -> [w237 _]
                      frame "Closed" {
                        n93 = invoke class="VI" method="FP.Open"(reference=w237, error in=w238, "Activate"=TRUE, "State"=T9."Standard") -> (error out=w239:errorcluster)  [unwired: 1 in, 4 out]
                      }
                      frame Default {
                      }
                    }
                  }
                  frame "Close" {
                    n94 = property class="VI"(reference=w245, error in=w247) -> (reference out=w244:refnum<vi>, error out=w246:errorcluster, "FP.State"=w243:T9)
                    n95 = case shown="Default" w243 {
                      tunnel: [w249 w252] -> w248
                      tunnel: w246 -> [w249 w251]
                      tunnel: w244 -> [_ w250]
                      frame "Invalid", "Closed" {
                      }
                      frame Default {
                        n96 = invoke class="VI" method="FP.Close"(reference=w250, error in=w251) -> (error out=w252:errorcluster)  [unwired: 1 in, 2 out]
                      }
                    }
                  }
                }
              }
              frame condition #1 {
              }
            }
            n97 = call <vilib>:"Add State(s) to Queue__jki_lib_state_machine.vi"("State(s) in (\"\")"=w226) -> ("States Out"=w225:string)  [unwired: 14 in]
          }
          frame "---------- Macro ----------" {
            # "Do not put any code in this frame.\n(It is a separator no-op. You can make a copy of this frame to create a new Macro frame)"
            n98 = call <vilib>:"Add State(s) to Queue__jki_lib_state_machine.vi"("State(s) in (\"\")"=w258) -> ("States Out"=w257:string)  [unwired: 14 in]
          }
          frame "Macro: Initialize" {
            w261 = "UI: Initialize\n//UI: Front Panel State >> Open"  # UI: Initialize //UI: Front Panel State >> Open
            # "Initialization Macro\n(This is called once, when the VI starts)"
            n99 = call <vilib>:"Add State(s) to Queue__jki_lib_state_machine.vi"("State(s) in Front (\"\")"="Data: Initialize\nInitialize Core Data\nEvents: Register", "State(s) in (\"\")"="Process: Sync", "State(s) at Back (\"\")"=w261) -> ("States Out"=w260:string)  [unwired: 12 in]
            n100 = call <vilib>:"Add State(s) to Queue__jki_lib_state_machine.vi"("State(s) in Front (\"\")"=w260, "State(s) in (\"\")"=w267) -> ("States Out"=w266:string)  [unwired: 13 in]
          }
          frame "Macro: Exit" {
            # "Exit Macro\n(This is called once, when the VI exits)"
            n101 = Unbundle By Name(w272) -> ("Core.Close Panel on Exit?"=w278:bool)
            n102 = Select(t="//UI: Front Panel State >> Close", s=w278, f="") -> (s? t:f=w275:string)
            n103 = call <vilib>:"Add State(s) to Queue__jki_lib_state_machine.vi"("State(s) in Front (\"\")"="Data: Cleanup\nEvents: Unregister\nProcess: Self Terminate", "State(s) in (\"\")"="Process: Sync", "State(s) at Back (\"\")"="Exit") -> ("States Out"=w269:string)  [unwired: 12 in]
            n104 = call <vilib>:"Add State(s) to Queue__jki_lib_state_machine.vi"("State(s) in (\"\")"=w275, "State(s) at Back (\"\")"=w269) -> ("States Out"=w274:string)  [unwired: 13 in]
            n105 = call <vilib>:"Add State(s) to Queue__jki_lib_state_machine.vi"("State(s) in Front (\"\")"=w274, "State(s) in (\"\")"=w281) -> ("States Out"=w280:string)  [unwired: 13 in]
          }
          frame "---------- Process ----------" {
            # "Template Separator\n(You can make a copy of, or modify, this frame)"
            n106 = call <vilib>:"Add State(s) to Queue__jki_lib_state_machine.vi"("State(s) in (\"\")"=w286) -> ("States Out"=w285:string)  [unwired: 14 in]
          }
          frame "Process: Sync" {
            n107 = Unbundle By Name(w294) -> ("Self Reference"=w290:refnum<class "SR7220 UI.lvclass">)
            n108 = call <vilib>:"WaitOnProcessSync.vi"("error in (no error)"=w289, "SMO"=w290) -> ("error out"=w288:errorcluster, "Don't run?"=w293:bool)  [unwired: 7 in, 1 out]
            n109 = Select(t="Data: Cleanup\nEvents: Unregister\nExit", s=w293, f="") -> (s? t:f=w287:string)
            n110 = call <vilib>:"Add State(s) to Queue__jki_lib_state_machine.vi"("State(s) in Front (\"\")"=w287, "State(s) in (\"\")"=w297) -> ("States Out"=w296:string)  [unwired: 13 in]
          }
          frame "Process: Self Terminate" {
            n111 = Unbundle By Name(w299) -> ("Self Reference"=w298:refnum<class "SR7220 UI.lvclass">)
            n112 = call <vilib>:"SelfTerminate.vi"("error in (no error)"=w301, "SMO in"=w298) -> ("error out"=w300:errorcluster)  [unwired: 8 in, 1 out]
            n113 = call <vilib>:"Add State(s) to Queue__jki_lib_state_machine.vi"("State(s) in (\"\")"=w304) -> ("States Out"=w303:string)  [unwired: 14 in]
          }
          frame "---------- Events ----------" {
            # "Template Separator\n(You can make a copy of, or modify, this frame)"
            n114 = call <vilib>:"Add State(s) to Queue__jki_lib_state_machine.vi"("State(s) in (\"\")"=w309) -> ("States Out"=w308:string)  [unwired: 14 in]
          }
          frame "Events: Register" {
            # "Expand to add\nmore events"
            # "Base Class Protected Events"
            n115 = Unbundle By Name(w320) -> ("Self Reference"=w313:refnum<class "SR7220 UI.lvclass">, "Instrument"=w312:refnum<class "Instrument.lvclass">)
            n116 = call <vilib>:"GetProtectedEvents.vi"("SMO"=w313) -> ("error out"=w314:errorcluster, "SMO Protected Events"=w318:T14)  [unwired: 8 in, 1 out]
            n117 = call "Instrument.GetPublicEvents.vi"("Instrument"=w312) -> ("error out"=w310:errorcluster, "Instrument Public Events"=w311:T15)  [unwired: 8 in, 1 out]
            n118 = register-events(w318, w311) -> (reference out=w319:refnum<event-registration>, error out=w316:errorcluster)  [unwired: 2 in]
            n119 = Merge Errors(w310, w317, w316, w314) -> (w315:errorcluster)
            n120 = call <vilib>:"Add State(s) to Queue__jki_lib_state_machine.vi"("State(s) in (\"\")"=w322) -> ("States Out"=w321:string)  [unwired: 14 in]
          }
          frame "Events: Unregister" {
            n121 = Unregister For Events(event registration refnum=w325, error in=w324) -> (error out=w323:errorcluster)
            n122 = call <vilib>:"Add State(s) to Queue__jki_lib_state_machine.vi"("State(s) in (\"\")"=w328) -> ("States Out"=w327:string)  [unwired: 14 in]
          }
          frame "---------- Action ----------" {
            n123 = Unbundle By Name(w331) -> ("Self Reference"=w329:refnum<class "SR7220 UI.lvclass">)
            n124 = Bundle By Name(cluster=w331, "Self Reference"=w329) -> (w330:T12)
            n125 = call <vilib>:"Add State(s) to Queue__jki_lib_state_machine.vi"("State(s) in (\"\")"=w335) -> ("States Out"=w334:string)  [unwired: 14 in]
          }
          frame "Action: Notify UI Closed" {
            # "Notify that the UI has been closed"
            n126 = Unbundle By Name(w338) -> ("Self Reference"=w339:refnum<class "SR7220 UI.lvclass">)
            n127 = call <vilib>:"Hide.vi"("error in (no error)"=w337, "SMO.UI"=w339) -> ("error out"=w336:errorcluster)  [unwired: 8 in, 1 out]
            n128 = call <vilib>:"Add State(s) to Queue__jki_lib_state_machine.vi"("State(s) in (\"\")"=w342) -> ("States Out"=w341:string)  [unwired: 14 in]
          }
          frame "Action: Update Front Panel" {
            # "do this way to have nicer UI or only display what you want"
            # "typedef from Child Instrument"
            n129 = Unbundle By Name(w352) -> ("getAll"=w351:variant)
            n130 = Variant To Data(error in=w350, type=dbl[] [], Variant=w351) -> (data=w347:dbl[], error out=w349:errorcluster)
            n131 = Index Array(array=w347) -> (element #1=→"Numeric" →"Slide":dbl, element #2=→"Numeric 2" →"Slide 2":dbl, element #3=→"Numeric 3" →"Slide 3":dbl, element #4=→"Numeric 4" →"Slide 4":dbl)  [unwired: 4 in]
            n132 = call <vilib>:"Add State(s) to Queue__jki_lib_state_machine.vi"("State(s) in (\"\")"=w355) -> ("States Out"=w354:string)  [unwired: 14 in]
          }
          frame "Action: Config" {
            n133 = Unbundle By Name(w363) -> ("Instrument"=w356:refnum<class "Instrument.lvclass">, "Data"=w358:variant)
            n134 = Bundle By Name(cluster=T10 {"Message"={"Command"="", "Data"=variant}, "Message ID"=0} ("SendMessage"), "Message.Data"=w358, "Message.Command"=w357) -> (w359:T10)
            n135 = call "Instrument.SendMessage.vi"("error in (no error)"=w362, "SendMessage"=w359, "Instrument"=w356) -> ("error out"=w361:errorcluster)  [unwired: 7 in, 1 out]
            n136 = call <vilib>:"Add State(s) to Queue__jki_lib_state_machine.vi"("State(s) in (\"\")"=w366) -> ("States Out"=w365:string)  [unwired: 14 in]
          }
        }
      }
    }
    frame Error {
    }
  }
  n137 = call-parent "Process.vi"("error in (no error)"=w8, "SMO.UI"=w7) -> ("error out"=w5:errorcluster, "SMO.UI out"=→"Example Instrument UI out":refnum<class "SR7220 UI.lvclass">)  [unwired: 8 in]
  n138 = Merge Errors(w5, w4) -> (→"error out":errorcluster)
